vi "Datasheet Generate Table Label.vi"(11 "Column Data":T1[](array[typedef])) -> (2 "Comma Label Row":string, 3 "HTM Table Row":string)   [LabVIEW 2011]
uses:
  Column Data.ctl
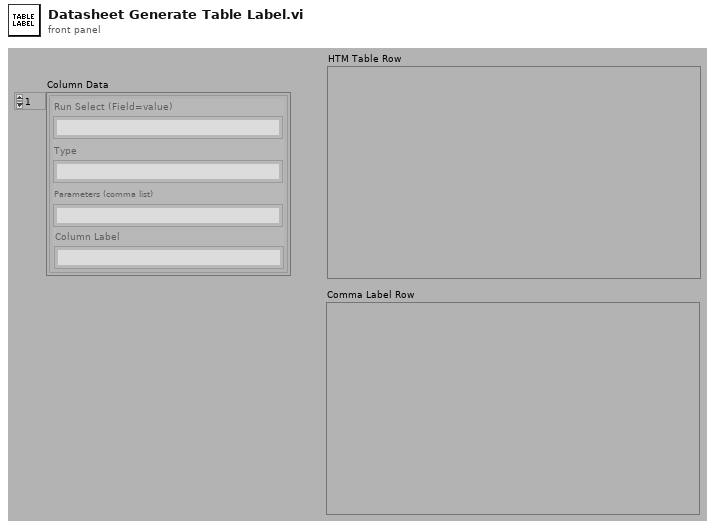
[diagram p1: front panel]
types:
  T1 = typedef "Column Data.ctl" = cluster{"Run Select (Field=value)":string, "Type":string, "Parameters (comma list)":string, "Column Label":string}
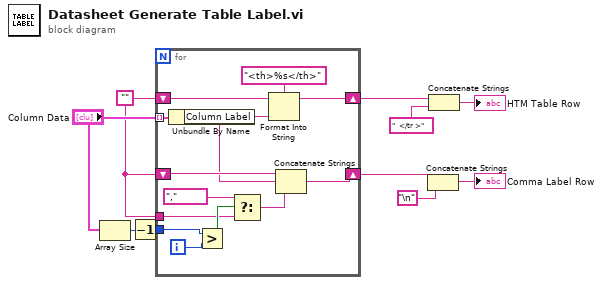
[diagram p0: block diagram]
diagram:
  w2 = ""
  n1 = Array Size(array="Column Data") -> (size(s)=w3:i32)
  n2 = Decrement(x=w3) -> (x-1=w1:i32)
  n3 = for {
    shift-right: [w22] -> w10
    shift-left: w2 -> [w21]
    tunnel: "Column Data" -> [w20] mode=indexing
    shift-right: [w17] -> w7
    shift-left: w2 -> [w19]
    tunnel: w1 -> [w14]
    tunnel: w2 -> [w11]
    i -> [w13]
    n4 = Unbundle By Name(w20) -> ("Column Label"=w18:string)
    n5 = Greater?(x=w14, y=w13) -> (0:w12:bool)
    n6 = Select(t="," ("format string"), s=w12, f=w11) -> (s? t:f=w16:string)
    n7 = Format Into String(format string="<th>%s</th>", initial string=w21, w18) -> (resulting string=w22:string)  [unwired: 1 in, 1 out]
    n8 = Concatenate Strings(w19, w18, w16) -> (w17:string)
  }
  n9 = Concatenate Strings(w7, "\n") -> (→"Comma Label Row":string)
  n10 = Concatenate Strings(w10, "  </tr >" ("format string")) -> (→"HTM Table Row":string)
